vi "GC Vacuum - Step 1.vi"(7 "Step":i32, 8 "error in":errorcluster, 9 "Test Results In":T8, 10 "Gas":T1, 11 "GC Configuration":T2) -> (0 "error out":errorcluster, 1 "Test Results Out":T8, 2 "Gas Out":T1 caption="Gas", 3 "GC Configuration Out":T2)   [LabVIEW 2015]
uses:
  Controls/Test Information.ctl
  Controls/Vacuum Test.ctl
  Controls/Test Timing.ctl
  Controls/Vaccum Thresholds.ctl
  Controls/Helium Test.ctl
  Controls/Helium Thresholds.ctl
  CAN Communication/Gas/Typedefs/Session Handle.ctl
  CAN Communication/Gas/Gas.lvclass
  Controls/Test Results.ctl
  Controls/Step Result.ctl
  SubVIs/Timing/Timing.lvlib
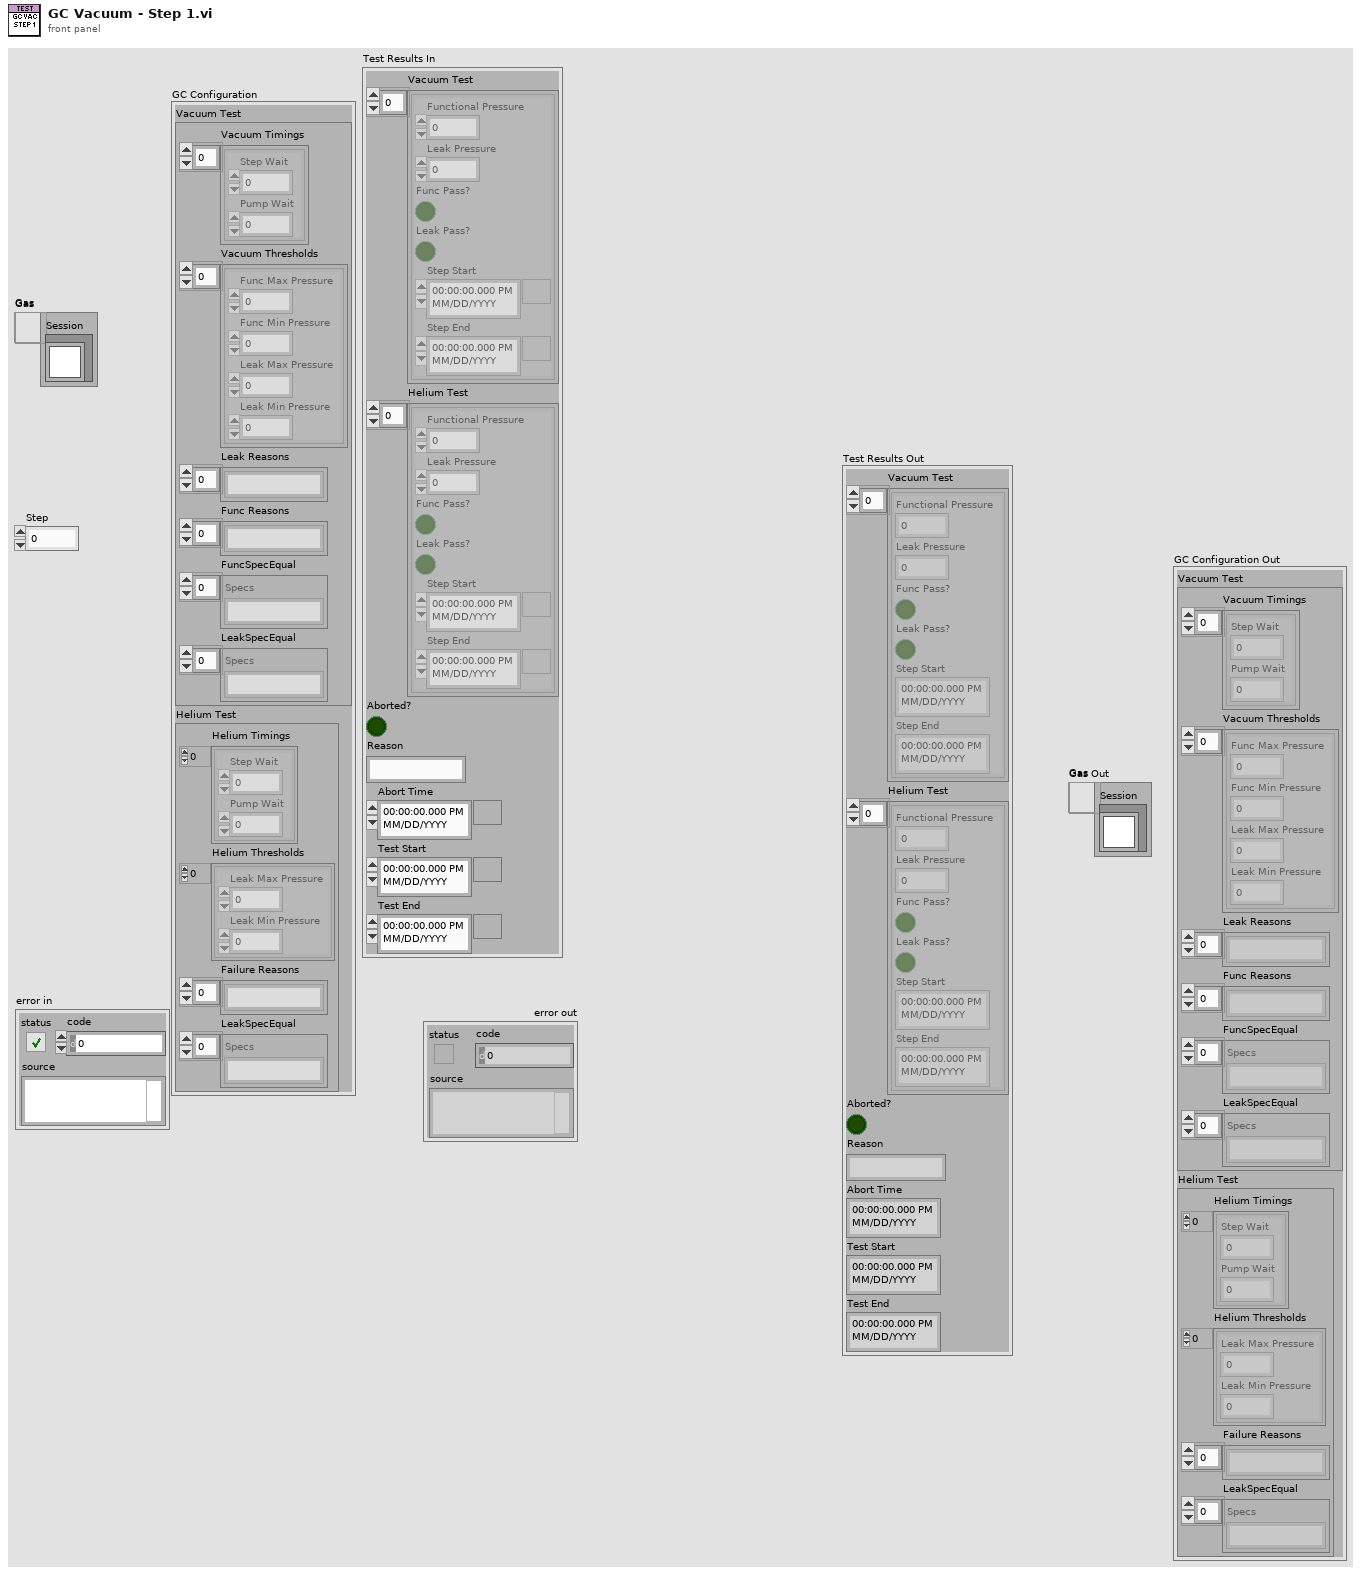
[diagram p1: front panel]
types:
  T1 = typedef "Gas.lvclass/Session Handle.ctl" = refnum<data-value>
  T2 = typedef "Test Information.ctl" = cluster{"Vacuum Test":T3, "Helium Test":T6}
  T3 = typedef "Vacuum Test.ctl" = cluster{"Vacuum Timings":T4[], "Vacuum Thresholds":T5[], "Leak Reasons":string[], "Func Reasons":string[], "FuncSpecEqual":string[], "LeakSpecEqual":string[]}
  T4 = typedef "Test Timing.ctl" = cluster{"Step Wait":dbl, "Pump Wait":dbl}
  T5 = typedef "Vaccum Thresholds.ctl" = cluster{"Func Max Pressure":dbl, "Func Min Pressure":dbl, "Leak Max Pressure":dbl, "Leak Min Pressure":dbl}
  T6 = typedef "Helium Test.ctl" = cluster{"Helium Timings":T4[], "Helium Thresholds":T7[], "Failure Reasons":string[], "LeakSpecEqual":string[]}
  T7 = typedef "Helium Thresholds.ctl" = cluster{"Leak Max Pressure":dbl, "Leak Min Pressure":dbl}
  T8 = typedef "Test Results.ctl" = cluster{"Vacuum Test":T9[], "Helium Test":T9[], "Aborted?":bool, "Reason":string, "Abort Time":timestamp, "Test Start":timestamp, "Test End":timestamp}
  T9 = typedef "Step Result.ctl" = cluster{"Functional Pressure":dbl, "Leak Pressure":dbl, "Func Pass?":bool, "Leak Pass?":bool, "Step Start":timestamp, "Step End":timestamp}
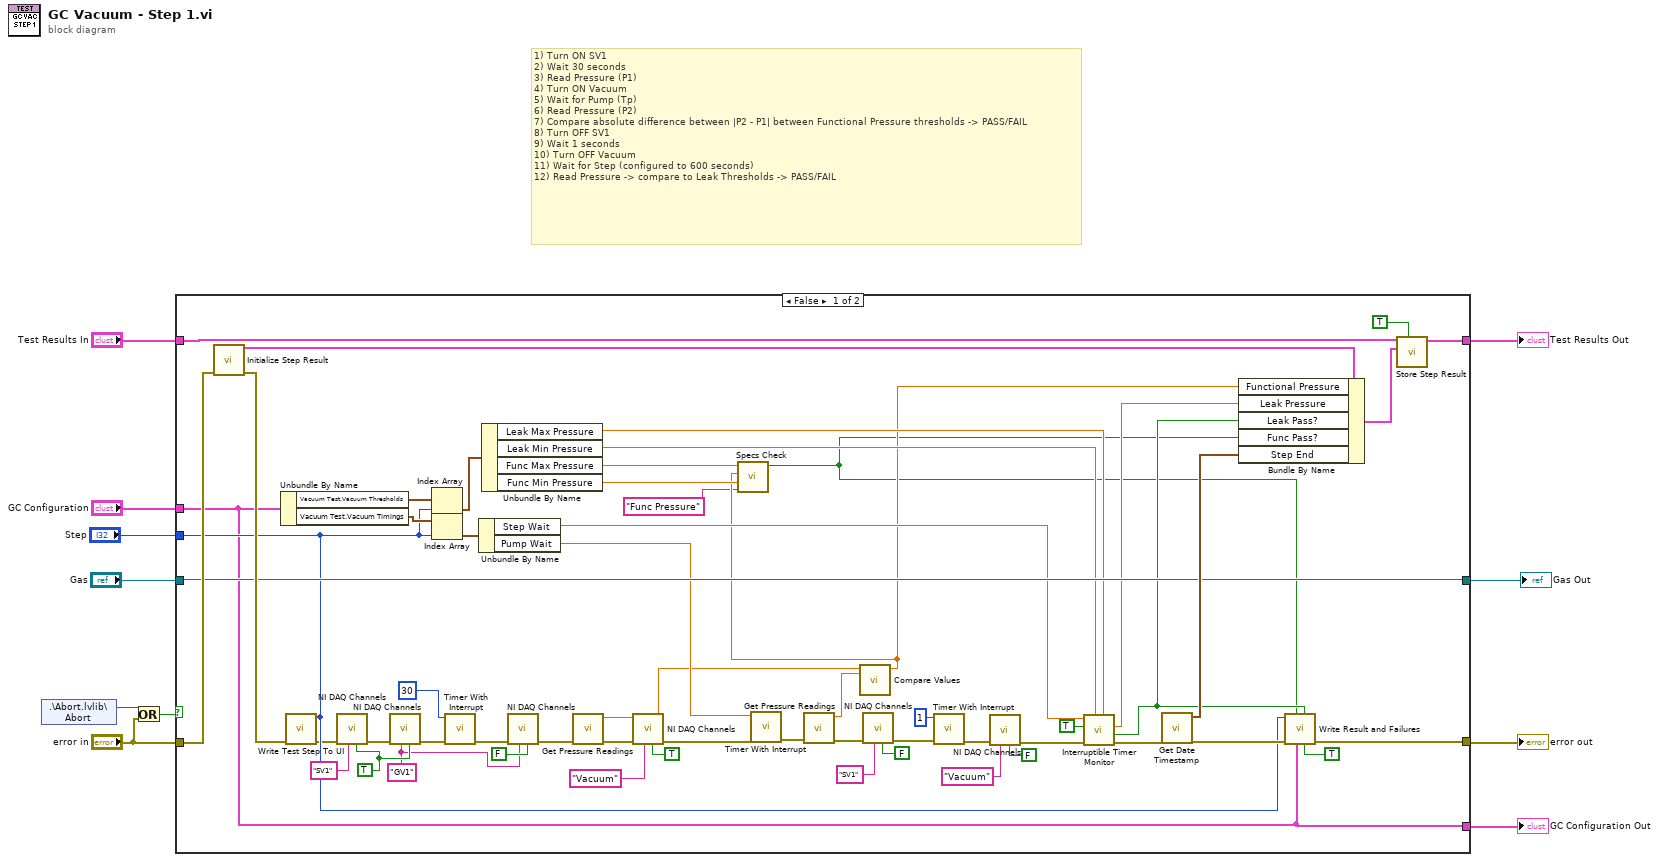
[diagram p0: block diagram]
diagram:
  # "1) Turn ON SV1\n2) Wait 30 seconds\n3) Read Pressure (P1)\n4) Turn ON Vacuum\n5) Wait for Pump (Tp)\n6) Read Pressure (P2)\n7) Compare absolute difference between |P2 - P1| between Functional Pressure thresholds -> PASS/FAIL\n8) Turn OFF SV1\n9) Wait 1 seconds\n10) Turn OFF Vacuum\n11) Wait for Step (configured to 600 seconds)\n12) Read Pressure -> compare to Leak Thresholds -> PASS/FAIL"
  n1 = shared-variable ".\\Abort.lvlib\\Abort"() -> (w10:bool)  [unwired: 1 in, 1 out]
  n2 = Or(x=w10, y="error in") -> (x .or. y?=w9:bool)
  n3 = case shown="False" w9 {
    tunnel: "error in" -> [w68 w71]
    tunnel: "Test Results In" -> [w65 w72]
    tunnel: [w66 w72] -> w7
    tunnel: [w49 w71] -> w6
    tunnel: "GC Configuration" -> [w47 w70]
    tunnel: "Step" -> [w48 _]
    tunnel: [w47 w70] -> w3
    tunnel: [w58 w69] -> w1
    tunnel: "Gas" -> [w58 w69]
    frame False {
      w21 = "GV1" ("Channel")
      w23 = TRUE ("State")
      n4 = call "Initialize Step Result.vi"("error in (no error)"=w68) -> ("error out"=w67:errorcluster, "New Step Result"=w64:T9)  [unwired: 8 in, 1 out]
      n5 = Unbundle By Name(w47) -> ("Vacuum Test.Vacuum Thresholds"=w61:T5[], "Vacuum Test.Vacuum Timings"=w60:T4[])
      n6 = call "Write Test Step To UI.vi"("error in (no error)"=w67, "Step"=w48) -> ("error out"=w45:errorcluster)  [unwired: 9 in]
      n7 = call "NI DAQ Channels.vi"("Control"=w23, "Channel"="SV1", "error in (no error)"=w45) -> ("error out"=w18:errorcluster)  [unwired: 7 in, 1 out]
      n8 = call "NI DAQ Channels.vi"("Control"=w23, "Channel"=w21, "error in (no error)"=w18) -> ("error out"=w17:errorcluster)  [unwired: 7 in, 1 out]
      n9 = Index Array(array=w61, index=w48) -> (element=w55:T5)
      n10 = Index Array(array=w60, index=w48) -> (element=w59:T4)
      n11 = call "Timer With Interrupt.vi"("error in (no error)"=w17, "Wait (s)"=30) -> ("error out"=w19:errorcluster)  [unwired: 7 in, 2 out]
      n12 = Unbundle By Name(w59) -> ("Step Wait"=w33:dbl, "Pump Wait"=w56:dbl)
      n13 = Unbundle By Name(w55) -> ("Leak Max Pressure"=w30:dbl, "Leak Min Pressure"=w31:dbl, "Func Max Pressure"=w16:dbl, "Func Min Pressure"=w15:dbl)
      n14 = call "NI DAQ Channels.vi"("Control"=FALSE, "Channel"=w21, "error in (no error)"=w19) -> ("error out"=w20:errorcluster)  [unwired: 7 in, 1 out]
      n15 = call "Get Pressure Readings.vi"("error in (no error)"=w20) -> ("error out"=w40:errorcluster, "NI-DAQ Pressure"=w52:dbl)  [unwired: 6 in, 3 out]
      n16 = call "NI DAQ Channels.vi"("Control"=TRUE ("State"), "Channel"="Vacuum", "error in (no error)"=w40) -> ("error out"=w39:errorcluster)  [unwired: 7 in, 1 out]
      n17 = call "Timer With Interrupt.vi"("error in (no error)"=w39, "Wait (s)"=w56) -> ("error out"=w54:errorcluster)  [unwired: 7 in, 2 out]
      n18 = call "Get Pressure Readings.vi"("error in (no error)"=w54) -> ("error out"=w43:errorcluster, "NI-DAQ Pressure"=w53:dbl)  [unwired: 6 in, 3 out]
      n19 = call "Compare Values.vi"("P2"=w53, "P1"=w52) -> ("Abs Diff"=w14:dbl)  [unwired: 9 in]
      n20 = call "Specs Check.vi"("parameter"="Func Pressure", "lower limit"=w15, "x"=w14, "upper limit"=w16) -> ("In Range?"=w13:bool)  [unwired: 6 in, 1 out]
      n21 = call "NI DAQ Channels.vi"("Control"=FALSE ("State"), "Channel"="SV1", "error in (no error)"=w43) -> ("error out"=w42:errorcluster)  [unwired: 7 in, 1 out]
      n22 = call "Timer With Interrupt.vi"("error in (no error)"=w42, "Wait (s)"=1) -> ("error out"=w37:errorcluster)  [unwired: 7 in, 2 out]
      n23 = call "NI DAQ Channels.vi"("Control"=FALSE ("State"), "Channel"="Vacuum", "error in (no error)"=w37) -> ("error out"=w35:errorcluster)  [unwired: 7 in, 1 out]
      n24 = call "Interruptible Timer Monitor.vi"("Max"=w30, "Min"=w31, "error in (no error)"=w35, "Update UI?"=TRUE, "Wait (s)"=w33) -> ("error out"=w34:errorcluster, "In Range?"=w28:bool, "Leak Rate"=w29:dbl)  [unwired: 2 in, 2 out]
      n25 = call "Get Date Timestamp.vi"("error in (no error)"=w34) -> ("error out"=w50:errorcluster, "current time"=w62:timestamp)  [unwired: 9 in]
      n26 = Bundle By Name(cluster=w64, "Functional Pressure"=w14, "Leak Pressure"=w29, "Leak Pass?"=w28, "Func Pass?"=w13, "Step End"=w62) -> (w63:T9)
      n27 = call "Write Result and Failures.vi"("Vacuum?"=TRUE, "Leak"=w28, "GC Configuration"=w47, "Func"=w13, "error in (no error)"=w50, "Step"=w48) -> ("error out"=w49:errorcluster)  [unwired: 5 in]
      n28 = call "Store Step Result.vi"("Vacuum?"=TRUE, "Step Result"=w63, "Test Results In"=w65) -> ("Test Results Out"=w66:T8)  [unwired: 8 in]
    }
    frame True {
    }
  }
  "error out" <- w6
  "Test Results Out" <- w7
  "GC Configuration Out" <- w3
  "Gas Out" <- w1
